vi "Get Mode.vi"(0 "object in":refnum<class "HPS-17000-PowerModule.lvclass">, 11 "Error In":errorcluster) -> (4 "object out":refnum<class "HPS-17000-PowerModule.lvclass">, 6 "Mode":string, 15 "Error Out":errorcluster)   [LabVIEW 2023, in "HPS-17000-PowerModule.lvlib" / "HPS-17000-PowerModule.lvclass"]
uses:
  HPS-17000-PowerModule.lvclass
  <instrlib>/HPS-17000/Internal/Get Mode Multi.vi
  HPS-17000-PowerModule.lvclass/HPS-17000-PowerModule.ctl
  <instrlib>/HPS-17000/HPS-17000.lvclass
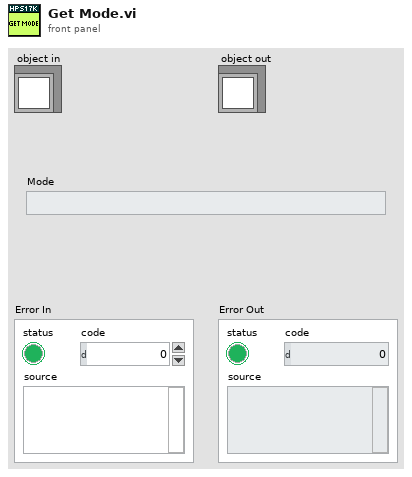
[diagram p1: front panel]
types:
  T1 = typedef "HPS-17000-PowerModule.lvlib/HPS-17000-PowerModule.lvclass/ObjectAttributes.ctl" = cluster{"JSON Config Path":path, "Configuration":T2, "GM ID":string, "HPS17000 Refs":refnum<class "HPS-17000.lvclass">[], "connected":bool, "reserved":bool, "events":T4, "nibatterycycler_grpc_Setpoint":T5, "last timestamp":i64, "mode":T6, "range":T7, "measurement array":T8[], "measurement stream":bool, "setpoint stream":bool}
  T2 = typedef "HPS-17000-PowerModule.lvlib/HPS-17000-PowerModule.lvclass/Configuration.ctl" = cluster{"TSN NIC IP Address":string, "HPS17000 IP Addresses":string[], "HPS Topology":enum16{"SINGLE", "MULTI"}, "Setpoint Stream Config":T3, "Measurement Array Size":i32}
  T3 = typedef "Cycler.lvclass/Setpoint Stream Basic Config.ctl" = cluster{"local address":string, "receiver port":u16}
  T4 = typedef "HPS-17000.lvclass/Multi-Cycler Events.ctl" = cluster{"heartbeats events":refnum<user-event>[], "faults events":refnum<user-event>[], "network sync event":refnum<user-event>[], "setpoint status event":refnum<user-event>[]}
  T5 = typedef "NI_BC_client.lvlib/nibatterycycler_grpc_Setpoint.ctl" = cluster{"voltage":sgl, "current":sgl, "min_power":sgl, "max_power":sgl, "resistance":sgl}
  T6 = typedef "HPS-17000-PowerModule.lvlib/HPS-17000-PowerModule.lvclass/Mode.ctl" = u16
  T7 = typedef "PowerModuleInterface.lvlibp/PowerModuleInterface.lvclass/Range.ctl" = cluster{"Current Max (A)":dbl, "Current Min (A)":dbl, "Voltage Max (V)":dbl, "Voltage Min (V)":dbl}
  T8 = typedef "PowerModuleInterface.lvlibp/PowerModuleInterface.lvclass/Measurements.ctl" = cluster{"measured voltage (V)":dbl, "measured current (A)":dbl, "setpoint voltage (V)":dbl, "setpoint current (A)":dbl, "timestamp":dbl}
  T9 = typedef "HPS-17000.lvclass/Mode.ctl" = u8
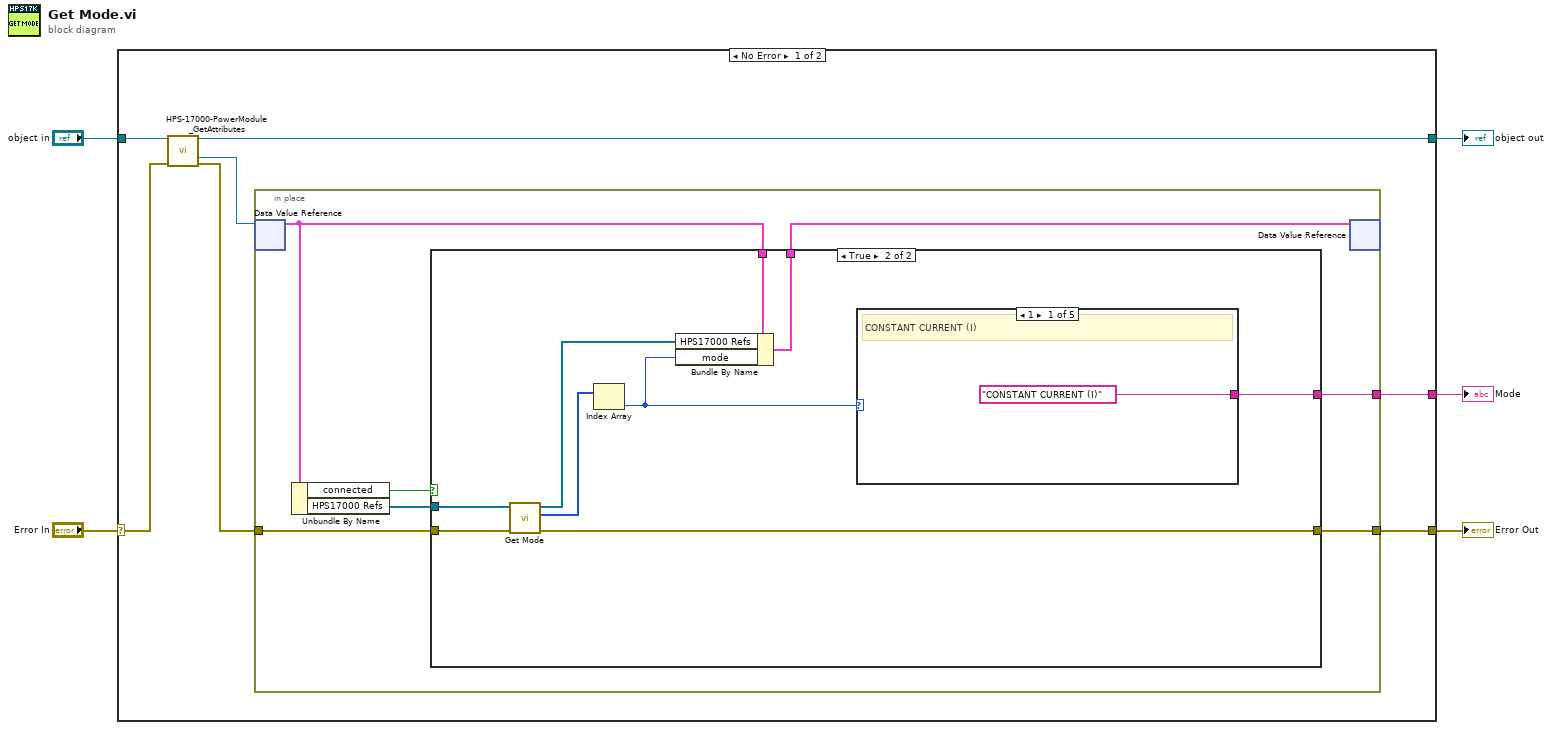
[diagram p0: block diagram]
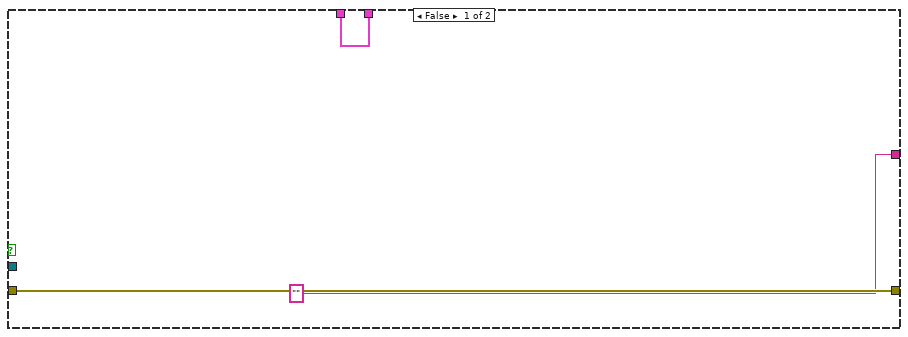
[diagram p2: hidden frame]
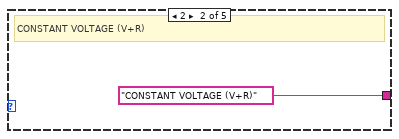
[diagram p3: hidden frame]
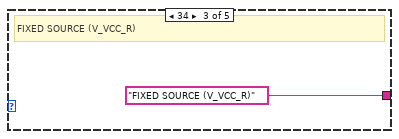
[diagram p4: hidden frame]
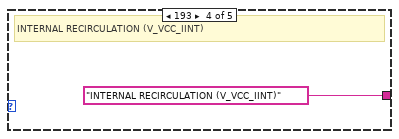
[diagram p5: hidden frame]
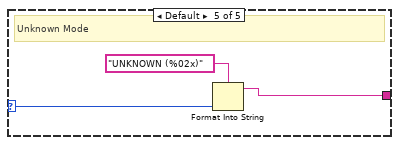
[diagram p6: hidden frame]
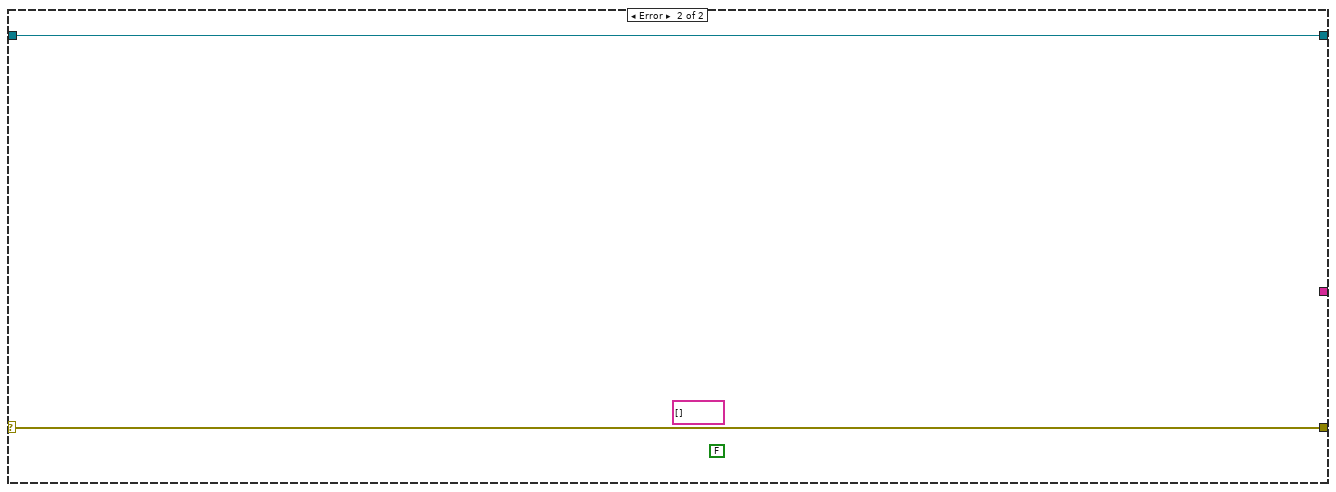
[diagram p7: hidden frame]
diagram:
  n1 = case shown="No Error" "Error In" {
    selector: "Error In" -> [w11 w39]
    tunnel: "object in" -> [w12 w40]
    tunnel: [w7 w40] -> w2
    tunnel: [w8 w39] -> w3
    tunnel: [w6 _] -> w1
    frame No Error {
      n2 = call "HPS-17000-PowerModule_GetAttributes.vi"("reference in"=w12, "Error In"=w11) -> ("reference out"=w7:refnum<class "HPS-17000-PowerModule.lvclass">, "DataRef"=w10:refnum<data-value>, "Error Out"=w9:errorcluster)  [unwired: 10 in, 1 out]
      n3 = in-place {
        in-place-border: w9 -> [w17]
        in-place-border: [w16] -> w8
        in-place-border: [w13] -> w6
        n4 = in-place-dvr #1(w10) -> (w18:T1)  [unwired: 1 out]
        n5 = Unbundle By Name(w18) -> ("connected"=w14:bool, "HPS17000 Refs"=w15:refnum<class "HPS-17000.lvclass">[])
        n6 = case shown="True" w14 {
          tunnel: [w22 w26] -> w19
          tunnel: w18 -> [w22 w31]
          tunnel: w17 -> [w21 w30]
          tunnel: [w21 w25] -> w16
          tunnel: w15 -> [_ w29]
          tunnel: ["" ("Mode") w24] -> w13
          frame False {
          }
          frame True {
            n7 = call-poly <instrlib>:"Get Mode.vi"("error in"=w30, "cycler refs in"=w29) -> ("error out"=w25:errorcluster, "mode"=w27:T9[], "cycler refs out"=w28:refnum<class "HPS-17000.lvclass">[])  [unwired: 6 in, 1 out]
            n8 = Index Array(array=w27) -> (element=w23:T9)  [unwired: 1 in]
            n9 = Bundle By Name(cluster=w31, "HPS17000 Refs"=w28, "mode"=w23) -> (w26:T1)
            n10 = case shown="1" w23 {
              selector: w23 -> [_ _ _ _ w37]
              tunnel: ["CONSTANT CURRENT (I)" ("Mode") "CONSTANT VOLTAGE (V+R)" ("Mode") "FIXED SOURCE (V_VCC_R)" ("Mode") "INTERNAL RECIRCULATION (V_VCC_IINT)" ("Mode") w36] -> w24
              frame 1 {
                # "CONSTANT CURRENT (I)"
              }
              frame 2 {
                # "CONSTANT VOLTAGE (V+R)"
              }
              frame 34 {
                # "FIXED SOURCE (V_VCC_R)"
              }
              frame 193 {
                # "INTERNAL RECIRCULATION (V_VCC_IINT)"
              }
              frame Default {
                # "Unknown Mode"
                n11 = Format Into String(format string="UNKNOWN (%02x)" ("Mode"), w37) -> (resulting string=w36:string)  [unwired: 2 in, 1 out]
              }
            }
          }
        }
        n12 = in-place-dvr #1(w19) -> ()  [unwired: 2 out]
      }
    }
    frame Error {
      (unwired) string[] []
      (unwired) FALSE
    }
  }
  "Error Out" <- w3
  "object out" <- w2
  "Mode" <- w1
